vi "gfitsio-read-image-subset-variant.vi"(4 "npixels (rest)":i32[](array[numeric]), 6 "fpixel (origin)":i32[](array[numeric]), 7 "inc (1)":i32[](array[numeric]), 8 "error in (no error)":errorcluster, 11 "gfits refnum":T1) -> (0 "error out":errorcluster, 2 "Variant":variant, 3 "dup gfits refnum":T1)   [LabVIEW 2019, in "gfitsio.lvlib"]
doc: "Read a rectangular subset of the FITS data array. <B>fpixel</B>, <b>npixels</b>, and <b>inc</b> must have the same number of elements as the image has dimensions. <b>fpixel</b> specifies the first pixel in the subset. <b>npixels</b> specifies the number of pixels to read along each image dimension, and should be at least 1 for each dimension. The number of elements greater than 1 in <b>npixels</b> determines the dimensionality of the resulting array, and should match the dimensions of the array returned by the particular instance of the polymorphic GFITSIO read function used. <b>inc</b> specifies the decimation to use along each dimension of the image. 2 will read every other pixel, 3 will read every third pixel, and so on. <B>fpixel</B>, <b>npixels</b>, and <b>inc</b> must be specified in ROW-MAJOR order, with the fastest changing dimension (NAXIS1) listed last and the slowest changing dimension listed first. The array that is returned will be structured according to <B>npixels</B>."
uses:
  gfitsio.lvlib
  gfitsio-refnum.ctl
  <vilib>/Utility/VariantDataType/MemoryInfo.ctl
  <vilib>/Utility/VariantDataType/MemoryType.ctl
  <vilib>/Utility/VariantDataType/VariantType.lvlib
  gfitsio.dll
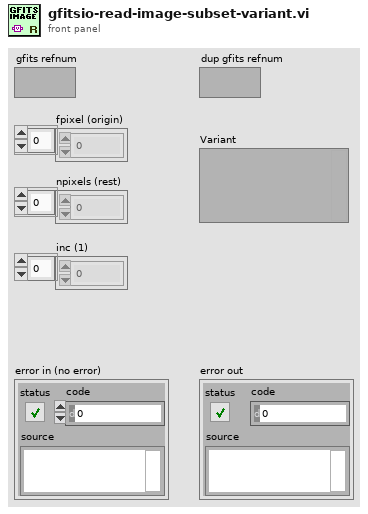
[diagram p1: front panel]
types:
  T1 = typedef "gfitsio.lvlib/gfitsio-refnum.ctl" = refnum<k1>
  T2 = typedef "gfitsio.lvlib/cfitsio-datatypes.ctl" = i32
  T3 = typedef "VariantType.lvlib/MemoryInfo.ctl" = cluster{"Type":T4, "Size":u32}
  T4 = typedef "VariantType.lvlib/MemoryType.ctl" = enum16{"Variable", "Fixed", "Bounded"}
  T5 = enum16{"big-endian, network order", "native, host order", "little-endian"}
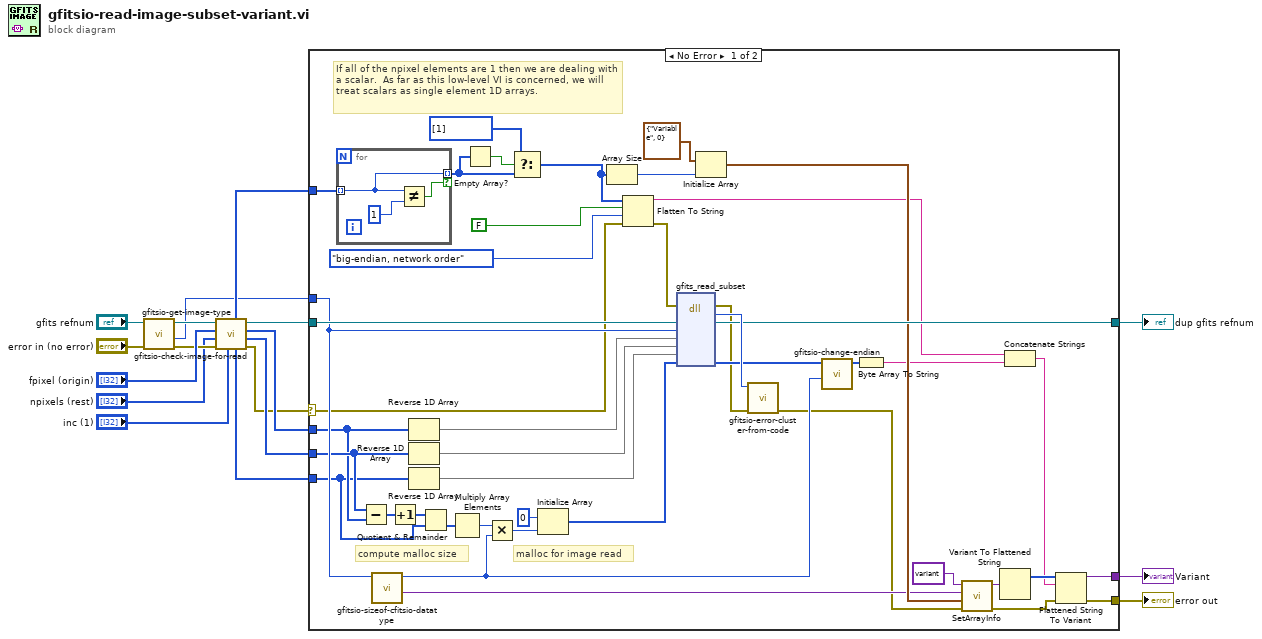
[diagram p0: block diagram]
diagram:
  n1 = call "gfitsio-get-image-type.vi"("error in (no error)"="error in (no error)", "gfits refnum"="gfits refnum") -> ("error out"=w4:errorcluster, "cfitsio datatype"=w1:T2, "dup gfits refnum"=w5:T1)  [unwired: 6 in, 1 out]
  n2 = call "gfitsio-check-image-for-read.vi"("inc"="inc (1)", "error in (no error)"=w4, "npixels"="npixels (rest)", "fpixel"="fpixel (origin)", "gfits refnum"=w5) -> ("error out"=w9:errorcluster, "lpixel out"=w14:i32[], "fpixel out"=w13:i32[], "dup gfits refnum"=w8:T1, "inc out"=w11:i32[], "npixels out"=w2:i32[])  [unwired: 1 in]
  n3 = case shown="No Error" w9 {
    selector: w9 -> [w37 w65]
    tunnel: [w28 w65] -> w16
    tunnel: w8 -> [w60 w66]
    tunnel: [w59 w66] -> w15
    tunnel: w13 -> [w20 _]
    tunnel: w14 -> [w21 _]
    tunnel: w11 -> [w19 _]
    tunnel: w1 -> [w55 _]
    tunnel: w2 -> [w45 _]
    tunnel: [w32 _] -> w17
    frame No Error {
      # "malloc for image read"
      # "compute malloc size"
      # "If all of the npixel elements are 1 then we are dealing with a scalar.  As far as this low-level VI is concerned, we will treat scalars as single element 1D arrays."
      n4 = for {
        tunnel: w45 -> [w63] mode=indexing
        tunnel: [w63] -> w26 mode=indexing if=w62
        n5 = Not Equal?(x=w63, y=1) -> (x != y?=w62:bool)
      }
      n6 = Subtract(x=w21, y=w20) -> (x-y=w23:i32[])
      n7 = call "gfitsio-sizeof-cfitsio-datatype.vi"("cfitsio datatype"=w55) -> ("Variant datatype"=w33:variant, "size (bytes)"=w50:i32)  [unwired: 8 in, 1 out]
      n8 = Increment(x=w23) -> (x+1=w22:i32[])
      n9 = Reverse 1D Array(array=w20) -> (reversed array=w56:i32[])
      n10 = Reverse 1D Array(array=w21) -> (reversed array=w57:i32[])
      n11 = Reverse 1D Array(array=w19) -> (reversed array=w58:i32[])
      n12 = Quotient & Remainder(x=w22, y=w19) -> (floor(x/y)=w18:i32[])  [unwired: 1 out]
      n13 = Multiply Array Elements(1:w18) -> (0:w49:i32)
      n14 = Empty Array?(array=w26) -> (empty?=w27:bool)
      n15 = Multiply(x=w49, y=w50) -> (x*y=w53:i32)
      n16 = Select(t=i32[] [1], s=w27, f=w26) -> (s? t:f=w24:i32[])
      n17 = Initialize Array(u8 0 ("X"), w53) -> (w52:u8[])
      n18 = Array Size(array=w24) -> (size(s)=w40:i32)
      n19 = Flatten To String(anything=w24, prepend array or string size? (T)=FALSE ("data includes array or string size? (T)"), byte order (0:big-endian, network order)=T5."big-endian, network order", error in (no error)=w37) -> (data string=w38:string, error out=w36:errorcluster)  [unwired: 1 out]
      n20 = dll-call lib="C:/Users/ggatling/local/GFITSIO/gfitsio/gfitsio.dll" fn="gfits_read_subset"(error in=w36, "handle"=w60, "datatype"=w55, "fpixel"=w56, "lpixel"=w57, "inc"=w58, "array"=w52) -> (error out=w35:errorcluster, "return type"=w61:i32, "handle"=w59:T1, "array"=w51:u8[])  [unwired: 6 in, 1 out]
      n21 = Initialize Array(T3 {"Type"=enum."Variable", "Size"=0} ("MemoryType"), w40) -> (w44:T3[])
      n22 = call "gfitsio-error-cluster-from-code.vi"("error in (no error)"=w35, "error code"=w61) -> ("error out"=w30:errorcluster)  [unwired: 9 in]
      n23 = call "gfitsio-change-endian.vi"("word size (bytes)"=w50, "data in"=w51) -> ("data out"=w48:u8[])  [unwired: 9 in]
      n24 = Byte Array To String(unsigned byte array=w48) -> (string=w39:string)
      n25 = call <vilib>:"SetArrayInfo.vi"("error in (no error)"=w30, "Array Lengths"=w44, "Array Element"=w33, "Variant"=variant(u8[] []) ("variant 2")) -> ("error out"=w29:errorcluster, "Variant Out"=w41:variant)  [unwired: 6 in]
      n26 = Variant To Flattened String(Variant=w41) -> (1:w42:i16[])  [unwired: 1 out]
      n27 = Concatenate Strings(w38, w39) -> (w34:string)
      n28 = Flattened String To Variant(4:w29, 6:w34, 7:w42) -> (0:w28:errorcluster, 3:w32:variant)
    }
    frame Error {
    }
  }
  "Variant" <- w17
  "error out" <- w16
  "dup gfits refnum" <- w15
